vi "TrajGetAverage.vi"(8 "error in (no error)":errorcluster, 11 "ForceField in":refnum<class "ForceField.lvclass">) -> (0 "error out":errorcluster, 2 "Ankle Traj Ave":dbl[][](array[numeric]), 3 "ForceField out":refnum<class "ForceField.lvclass">)   [LabVIEW 2016, in "ForceField.lvclass"]
uses:
  ForceField.lvclass
  ForceField.lvclass/ForceField.ctl
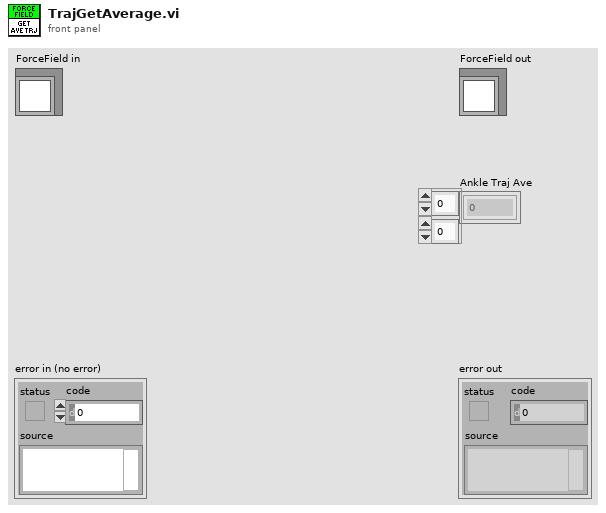
[diagram p1: front panel]
types:
  T1 = typedef "ForceField.lvclass/AnkleTrajPt.ctl" = cluster{"P1":dbl[], "P2":dbl[], "P1-P2":dbl[], "(P1-P2)^2":dbl}
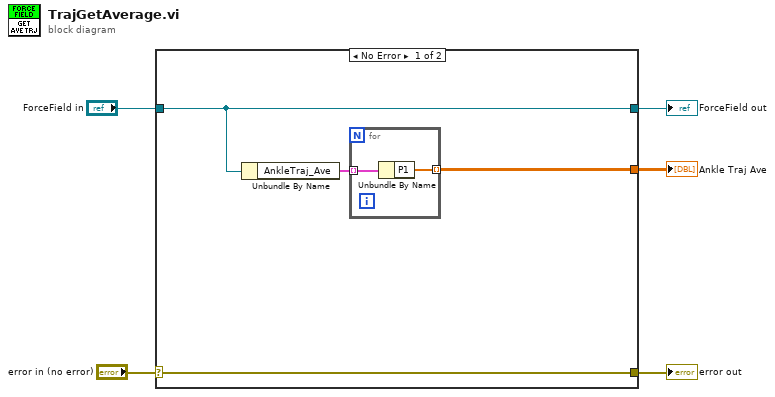
[diagram p0: block diagram]
diagram:
  n1 = case shown="No Error" "error in (no error)" {
    selector: "error in (no error)" -> [w9 w13]
    tunnel: [w9 w13] -> w4
    tunnel: [w8 w12] -> w2
    tunnel: "ForceField in" -> [w8 w12]
    tunnel: [w6 _] -> w1
    frame No Error {
      n2 = Unbundle By Name(w8) -> ("AnkleTraj_Ave"=w7:T1[])
      n3 = for {
        tunnel: w7 -> [w11] mode=indexing
        tunnel: [w10] -> w6 mode=indexing
        n4 = Unbundle By Name(w11) -> ("P1"=w10:dbl[])
      }
    }
    frame Error {
    }
  }
  "error out" <- w4
  "ForceField out" <- w2
  "Ankle Traj Ave" <- w1
